vi "sub_read_LAPD.vi"() -> (0 "data":dbl format="%_6g")   [LabVIEW 2009]
uses:
  <vilib>/ULx/Read.llb/ULx Read (Analog DBL 1Chan 1Samp).vi
  <vilib>/ULx/Create Channel.llb/ULx Create Channel (AI-Voltage-Basic).vi
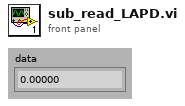
[diagram p1: front panel]
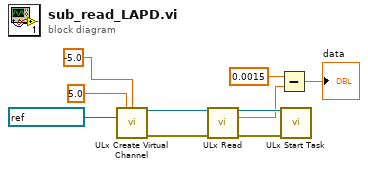
[diagram p0: block diagram]
diagram:
  n1 = call-poly <vilib>:"ULx Create Virtual Channel.vi"("maximum value"=5.0, "minimum value"=-5.0, "physical channels"=refnum<k21> "Dev1/Ai0") -> ("task out"=w8:refnum<k24>, "error out"=w7:errorcluster)  [unwired: 11 in]
  n2 = call-poly <vilib>:"ULx Read.vi"("task in"=w8, "error in"=w7) -> ("task out"=w10:refnum<k24>, "data"=w3:dbl, "error out"=w9:errorcluster)  [unwired: 11 in]
  n3 = Subtract(x=0.0015, y=w3) -> (x-y=→"data":dbl)
  n4 = call <vilib>:"ULx Start Task.vi"("task in"=w10, "error in"=w9) -> ()  [unwired: 12 in, 2 out]
